vi "Module Init.vi"(8 "error in (no error)":errorcluster, 11 "GUIHandler in":refnum<class "GUIHandler.lvclass">) -> (0 "error out":errorcluster, 3 "GUIHandler out":refnum<class "GUIHandler.lvclass">)   [LabVIEW 2020, in "VolatusGUI.lvlib" / "GUIHandler.lvclass"]
uses:
  GUIHandler.lvclass
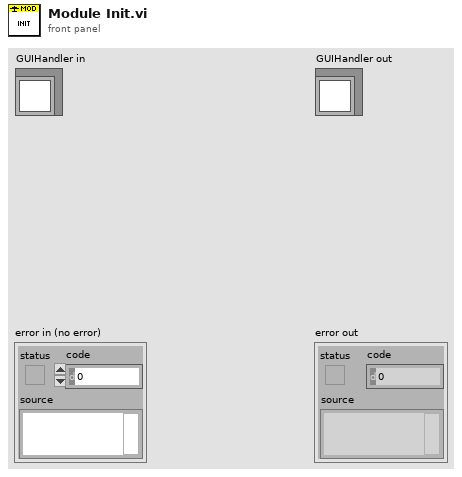
[diagram p1: front panel]
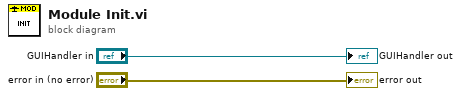
[diagram p0: block diagram]
diagram:
  "error out" <- "error in (no error)"
  "GUIHandler out" <- "GUIHandler in"
